vi "Zero Phase Filter (Cascade, CDB).vi"(10 "IIR Filter Cluster":T1 {"Forward Coefficients" format="%.4f"; "Reverse Coefficients" format="%.4f"}, 11 "X":cdb[](array[numeric])) -> (0 "error":i32, 3 "Filtered X":cdb[](array[numeric]))   [LabVIEW 2017, in "NI_AALBase.lvlib"]
doc: "Applies a zero phase filter to an input sequence <B>X</B>. Wire data to the <B>X</B> input to determine the polymorphic instance to use or manually select the instance."
uses:
  NI_AALBase.lvlib
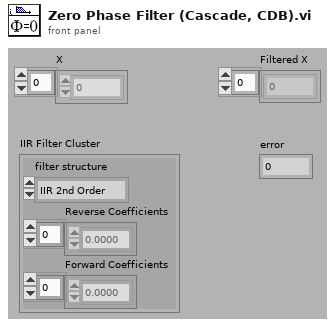
[diagram p1: front panel]
types:
  T1 = cluster{"filter structure":enum32{"IIR 2nd Order", "IIR 4th Order"}, "Reverse Coefficients":dbl[], "Forward Coefficients":dbl[]}
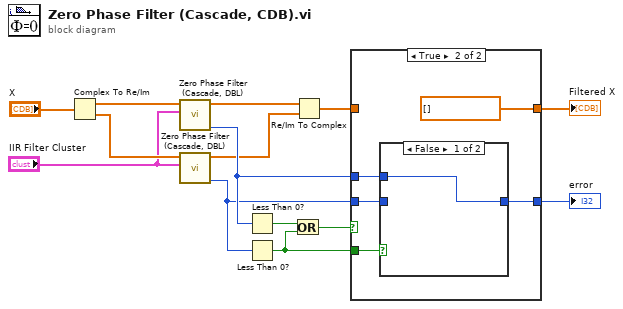
[diagram p0: block diagram]
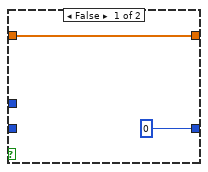
[diagram p2: hidden frame]
diagram:
  n1 = Complex To Re/Im(x + iy="X") -> (x=w9:dbl[], y=w8:dbl[])
  n2 = call "Zero Phase Filter (Cascade, DBL).vi"("IIR Filter Cluster"="IIR Filter Cluster", "X"=w9) -> ("error"=w6:i32, "Filtered X"=w3:dbl[])  [unwired: 8 in]
  n3 = call "Zero Phase Filter (Cascade, DBL).vi"("IIR Filter Cluster"="IIR Filter Cluster", "X"=w8) -> ("error"=w5:i32, "Filtered X"=w4:dbl[])  [unwired: 8 in]
  n4 = Less Than 0?(x=w6) -> (x < 0?=w11:bool)
  n5 = Less Than 0?(x=w5) -> (x < 0?=w14:bool)
  n6 = Or(x=w11, y=w14) -> (x .or. y?=w13:bool)
  n7 = Re/Im To Complex(1:w4, 2:w3) -> (0:w12:cdb[])
  n8 = case shown="True" w13 {
    tunnel: w12 -> [w16 _]
    tunnel: w14 -> [_ w21]
    tunnel: w5 -> [_ w20]
    tunnel: w6 -> [_ w19]
    tunnel: [0 ("error") w18] -> w1
    tunnel: [w16 cdb[] []] -> w2
    frame False {
    }
    frame True {
      n9 = case shown="False" w21 {
        tunnel: [w22 w23] -> w18
        tunnel: w20 -> [_ w23]
        tunnel: w19 -> [w22 _]
        frame False {
        }
        frame True {
        }
      }
    }
  }
  "Filtered X" <- w2
  "error" <- w1
